vi "Read Board To Display.vi"(8 "error in (no error)":errorcluster, 11 "Screen Interface in":refnum<class "Screen Interface.lvclass">) -> (0 "error out":errorcluster, 2 "Board To Display":u32[][](array[numeric]), 3 "Screen Interface out":refnum<class "Screen Interface.lvclass">)   [LabVIEW 2017, in "Screen Interface.lvlib" / "Screen Interface.lvclass"]
uses:
  Screen Interface.lvclass
  Screen Interface.lvclass/Screen Interface.ctl
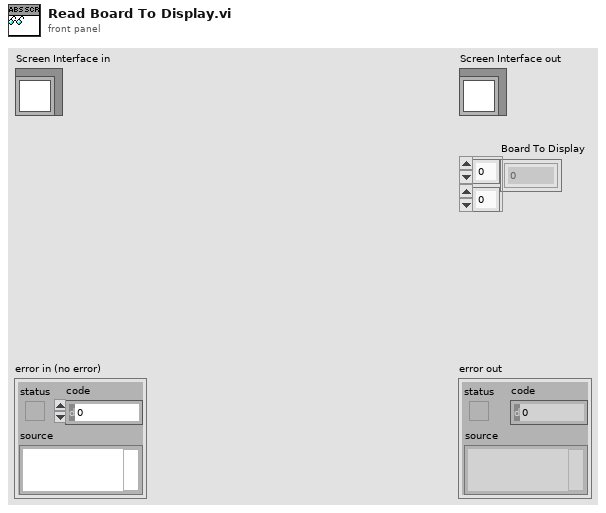
[diagram p1: front panel]
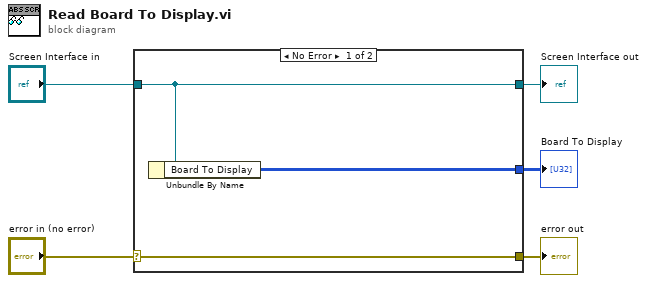
[diagram p0: block diagram]
diagram:
  n1 = case shown="No Error" "error in (no error)" {
    selector: "error in (no error)" -> [w8 w9]
    tunnel: [w8 w9] -> w4
    tunnel: [w7 w10] -> w2
    tunnel: "Screen Interface in" -> [w7 w10]
    tunnel: [w6 _] -> w1
    frame No Error {
      n2 = Unbundle By Name(w7) -> ("Board To Display"=w6:u32[][])
    }
    frame Error {
    }
  }
  "error out" <- w4
  "Screen Interface out" <- w2
  "Board To Display" <- w1
